vi "CRYDelete Data From Step.vi"(10 "Names In":string[](array[string]), 11 "Type In":enum16{"Curves", "Values", "Results", "WFM"}(ring)) -> (2 "No Names Out":string[](array[string]))   [LabVIEW 2013]
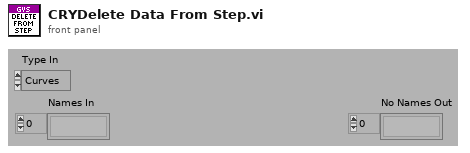
[diagram p1: front panel]
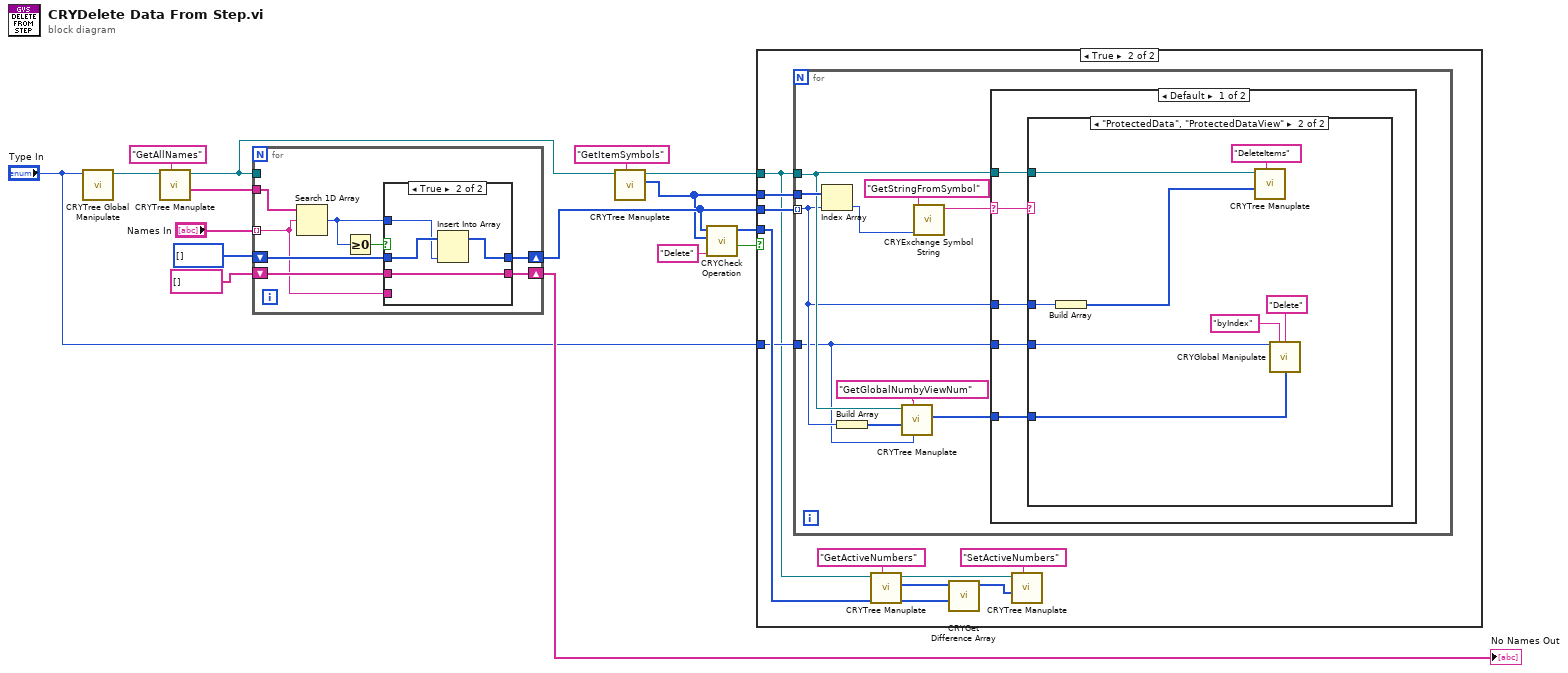
[diagram p0: block diagram]
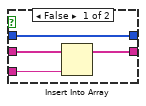
[diagram p2: hidden frame]
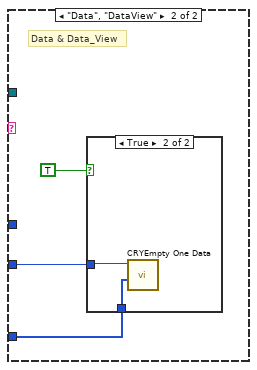
[diagram p5: hidden frame]
diagram:
  n1 = call "CRYTree Global Manipulate.vi"("Type In"="Type In") -> ("Tree/Curve Tree"=w1:refnum<vi>)  [unwired: 7 in, 3 out]
  n2 = call "CRYTree Manuplate.vi"("sAction"="GetAllNames", "Tree in"=w1) -> ("sData Out"=w7:string[], "Tree Out"=w4:refnum<vi>)  [unwired: 6 in, 2 out]
  n3 = for {
    tunnel: "Names In" -> [w18] mode=indexing
    tunnel: w4 -> [_]
    shift-right: [w21] -> w15
    shift-left: i32[] [] ("Value") -> [w22]
    shift-right: [w19] -> w10
    shift-left: string[] [] ("Names In") -> [w20]
    tunnel: w7 -> [w17]
    n4 = Search 1D Array(1D array=w17, element=w18) -> (index of element=w23:i32)  [unwired: 1 out]
    n5 = Greater Or Equal To 0?(x=w23) -> (x >= 0?=w24:bool)
    n6 = case shown="True" w24 {
      tunnel: w23 -> [_ w31]
      tunnel: [w28 w30] -> w21
      tunnel: w22 -> [w28 w32]
      tunnel: w20 -> [w27 w29]
      tunnel: [w26 w29] -> w19
      tunnel: w18 -> [w25 _]
      frame False {
        n7 = Insert Into Array(array=w27, new element=w25) -> (w26:string[])  [unwired: 1 in]
      }
      frame True {
        n8 = Insert Into Array(array=w32, new element=w31) -> (w30:i32[])  [unwired: 1 in]
      }
    }
  }
  "No Names Out" <- w10
  n9 = call "CRYTree Manuplate.vi"("sAction"="GetItemSymbols", "Tree in"=w4) -> ("nData Out"=w3:i32[], "Tree Out"=w5:refnum<vi>)  [unwired: 6 in, 2 out]
  n10 = call "CRYCheck Operation.vi"("Operation"="Delete", "Item Symbols In"=w3, "Index Array In"=w15) -> ("Operation ?"=w14:bool, "Array Out"=w16:i32[])  [unwired: 1 in, 6 out]
  n11 = case shown="True" w14 {
    tunnel: w5 -> [_ w36]
    tunnel: w15 -> [_ w42]
    tunnel: w3 -> [_ w41]
    tunnel: w16 -> [_ w40]
    tunnel: "Type In" -> [_ w39]
    frame False {
    }
    frame True {
      n12 = for {
        tunnel: w36 -> [w47]
        tunnel: w42 -> [w46] mode=indexing
        tunnel: w41 -> [w52]
        tunnel: w39 -> [w43]
        n13 = Index Array(array=w52, index=w46) -> (element=w50:i32)
        n14 = Build Array(w46) -> (w45:i32[])
        n15 = call "CRYTree Manuplate.vi"("Type"=w43, "sAction"="GetGlobalNumbyViewNum", "nData"=w45, "Tree in"=w47) -> ("nData Out"=w44:i32[])  [unwired: 4 in, 3 out]
        n16 = call "CRYExchange Symbol String.vi"("nData"=w50, "sAction"="GetStringFromSymbol") -> ("sData out"=w49:string)  [unwired: 8 in, 1 out]
        n17 = case shown="Default" w49 {
          selector: w49 -> [w54 _]
          tunnel: w46 -> [w56 _]
          tunnel: w47 -> [w57 _]
          tunnel: w43 -> [w55 w67]
          tunnel: w44 -> [w53 w66]
          frame Default {
            n18 = case shown="\"ProtectedData\", \"ProtectedDataView\"" w54 {
              tunnel: w57 -> [_ w64]
              tunnel: w56 -> [_ w63]
              tunnel: w55 -> [_ w58]
              tunnel: w53 -> [_ w60]
              frame Default {
                # "NoData"
                # "Nothing to do"
              }
              frame "ProtectedData", "ProtectedDataView" {
                n19 = Build Array(w63) -> (w61:i32[])
                n20 = call "CRYTree Manuplate.vi"("sAction"="DeleteItems", "nData"=w61, "Tree in"=w64) -> ()  [unwired: 5 in, 4 out]
                n21 = call "CRYGlobal Manipulate.vi"("Type"=w58, "sOption"="byIndex", "sAction"="Delete", "nData"=w60) -> ()  [unwired: 5 in, 7 out]
              }
            }
          }
          frame "Data", "DataView" {
            # "Data & Data_View"
            n22 = case shown="True" TRUE {
              tunnel: w67 -> [_ w70]
              tunnel: w66 -> [_ w69]
              frame False {
                # "There are some data\n not to delete."
                # "For the future"
              }
              frame True {
                n23 = call "CRYEmpty One Data.vi"("Index"=w69, "Type"=w70) -> ()  [unwired: 1 in, 9 out]
              }
            }
          }
        }
      }
      n24 = call "CRYTree Manuplate.vi"("sAction"="GetActiveNumbers", "Tree in"=w36) -> ("nData Out"=w35:i32[], "Tree Out"=w33:refnum<vi>)  [unwired: 6 in, 2 out]
      n25 = call "CRYGet Difference Array.vi"("Array 2"=w40, "Array 1"=w35) -> ("Diff Out"=w34:i32[])  [unwired: 3 in, 6 out]
      n26 = call "CRYTree Manuplate.vi"("sAction"="SetActiveNumbers", "nData"=w34, "Tree in"=w33) -> ()  [unwired: 5 in, 4 out]
    }
  }
